vi "GetClassHierarchy.vi"(1 "LabVIEWClass":refnum<vi>, 5 "error in (no error)":errorcluster) -> (15 "Classes":refnum<vi>[](array[refnum]), 17 "Level":i32[](array[numeric]), 19 "error out":errorcluster)   [LabVIEW 2020, in "G#IDE.lvlib" / "LibraryLib.lvlib"]
uses:
  <resource>/Framework/Providers/AddQ/G#IDE/support/LibraryLib/LibraryLib.lvlib
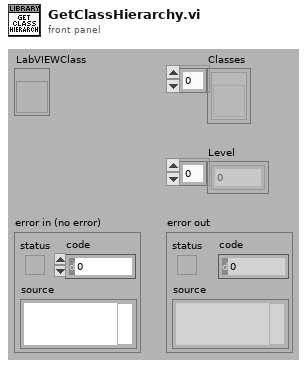
[diagram p1: front panel]
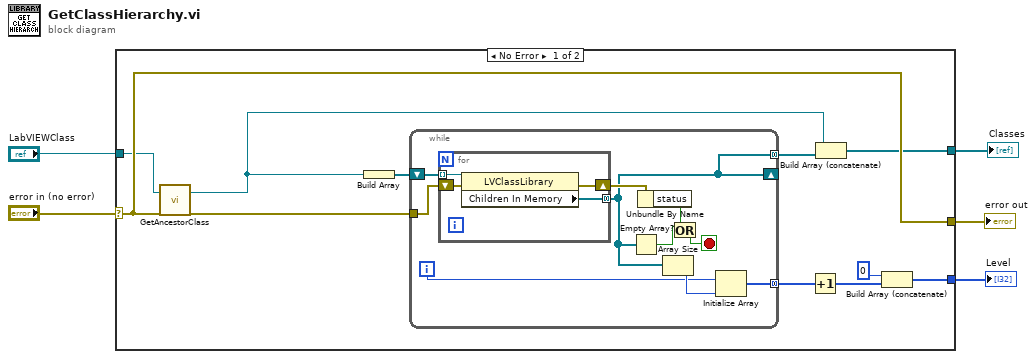
[diagram p0: block diagram]
diagram:
  n1 = case shown="No Error" "error in (no error)" {
    selector: "error in (no error)" -> [w16 w31]
    tunnel: [w16 w31] -> w5
    tunnel: "LabVIEWClass" -> [w14 _]
    tunnel: [w13 _] -> w2
    tunnel: [w9 _] -> w1
    frame No Error {
      n2 = call <resource>:"GetAncestorClass.vi"("LabVIEWClass"=w14, "error in (no error)"=w16) -> ("Ancestor"=w10:refnum<vi>, "error out"=w15:errorcluster)  [unwired: 16 in]
      n3 = Build Array(w10) -> (w11:refnum<vi>[])
      n4 = while {
        shift-right: [w20] -> _
        shift-left: w11 -> [w24]
        tunnel: w15 -> [w23]
        tunnel: [w20] -> w12 mode=concatenating
        tunnel: [w19] -> w7 mode=concatenating
        i -> [w17]
        stop <- w25 stop-if-true
        n5 = for {
          tunnel: w24 -> [w27] mode=indexing
          tunnel: [w28] -> w20 mode=concatenating
          shift-right: [w29] -> w22
          shift-left: w23 -> [w30]
          n6 = property class="LVClassLibrary"(reference=w27, error in=w30) -> (error out=w29:errorcluster, "Children In Memory"=w28:refnum<vi>[])  [unwired: 1 out]
        }
        n7 = Empty Array?(array=w20) -> (empty?=w21:bool)
        n8 = Unbundle By Name(w22) -> ("status"=w26:bool)
        n9 = Array Size(array=w20) -> (size(s)=w18:i32)
        n10 = Or(x=w21, y=w26) -> (x .or. y?=w25:bool)
        n11 = Initialize Array(w17, w18) -> (w19:i32[])
      }
      n12 = Increment(x=w7) -> (x+1=w6:i32[])
      n13 = Build Array (concatenate)(w10, w12) -> (w13:refnum<vi>[])
      n14 = Build Array (concatenate)(0, w6) -> (w9:i32[])
    }
    frame Error {
    }
  }
  "error out" <- w5
  "Classes" <- w2
  "Level" <- w1
